vi "Random-Graph(real time).vi"() -> ()   [LabVIEW 2014]
panel:
  out "Waveform Graph":dbl[](graph)
  in  "stop":bool
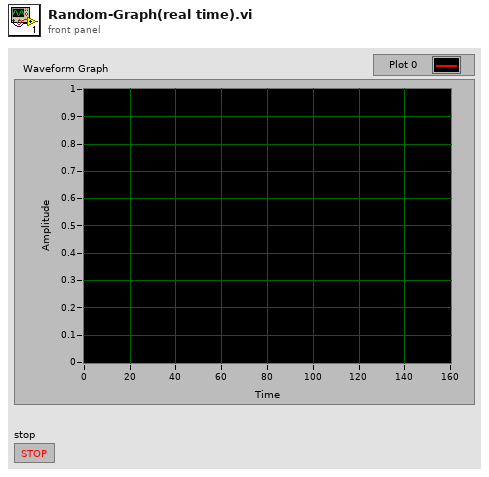
[diagram p1: front panel]
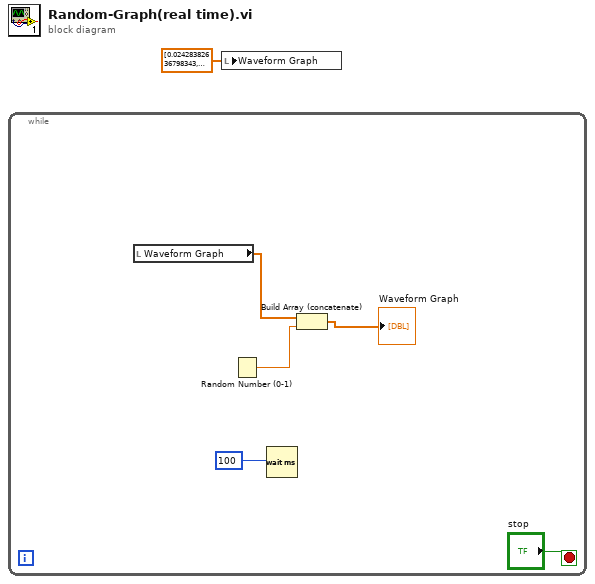
[diagram p0: block diagram]
diagram:
  n1 = while {
    stop <- "stop" stop-if-true
    n2 = local read "Waveform Graph"() -> (w4:dbl[])
    n3 = Random Number (0-1)() -> (number: 0 to 1=w3:dbl)
    n4 = Wait (ms)(milliseconds to wait=100) -> ()  [unwired: 1 out]
    n5 = Build Array (concatenate)(w4, w3) -> (→"Waveform Graph":dbl[])
  }
  n6 = local write "Waveform Graph"(dbl[] [0.02428382636798343, 0.8533299215121894, 0.8328407781087419, 0.5431372479534602, 0.9114287518707376, 0.6814595698667156, 0.20104495575424775, 0.3561782164733889, 0.7615327486071617, 0.8213640257337804, 0.5134674859212742, 0.9181006111664619, 0.5740434731710762, 0.830794799733662, 0.7360355066157889, 0.9323869653527188, 0.038262174853991304, 0.7536202371940048, 0.2949213461347502, 0.6249603852023782, 0.845131487260427, 0.30506983707623725, 0.8009282596387035, 0.7815108174904104, 0.2744320157491589, 0.42701608786091527] ("Waveform Graph")) -> ()
